vi "Test1.vi"   [LabVIEW 2020]
uses:
  MelsecMcNet/MelsecMcNet.lvclass
  lModbusRtu/ModbusRtu.lvclass
  InovanceTCP/InovanceModbusTcp.lvclass
  InovanceSerial/InovanceSerialModbusRtu.lvclass
  Abstract PLC Controler/Abs Controler.lvclass
  E:/Git/Libraries/develop/HslCommunication/Abstract PLC Controler/Abs Controler.lvclass
  E:/Git/Libraries/develop/HslCommunication/lModbusRtu/ModbusRtu.lvclass
  E:/Git/Libraries/develop/HslCommunication/MelsecMcNet/MelsecMcNet.lvclass
  E:/Git/Libraries/develop/HslCommunication/InovanceTCP/InovanceModbusTcp.lvclass
  E:/Git/Libraries/develop/HslCommunication/InovanceSerial/InovanceSerialModbusRtu.lvclass
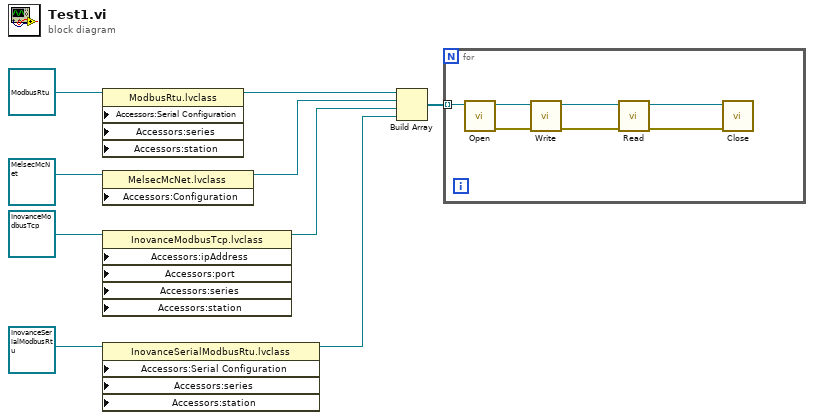
[diagram p0: block diagram]
diagram:
  n1 = property class="ModbusRtu.lvclass" props=["Accessors:Serial Configuration", "Accessors:series", "Accessors:station"](reference=refnum<class "ModbusRtu.lvclass"> refnum ("HslCommunication.lvlib:ModbusRtu.lvclass")) -> (reference out=w5:refnum<class "ModbusRtu.lvclass">)  [unwired: 4 in, 1 out]
  n2 = property class="MelsecMcNet.lvclass" props=["Accessors:Configuration"](reference=refnum<class "MelsecMcNet.lvclass"> refnum ("HslCommunication.lvlib:MelsecMcNet.lvclass")) -> (reference out=w3:refnum<class "MelsecMcNet.lvclass">)  [unwired: 2 in, 1 out]
  n3 = property class="InovanceModbusTcp.lvclass" props=["Accessors:ipAddress", "Accessors:port", "Accessors:series", "Accessors:station"](reference=refnum<class "InovanceModbusTcp.lvclass"> refnum ("HslCommunication.lvlib:InovanceModbusTcp.lvclass")) -> (reference out=w2:refnum<class "InovanceModbusTcp.lvclass">)  [unwired: 5 in, 1 out]
  n4 = property class="InovanceSerialModbusRtu.lvclass" props=["Accessors:Serial Configuration", "Accessors:series", "Accessors:station"](reference=refnum<class "InovanceSerialModbusRtu.lvclass"> refnum ("HslCommunication.lvlib:InovanceSerialModbusRtu.lvclass")) -> (reference out=w1:refnum<class "InovanceSerialModbusRtu.lvclass">)  [unwired: 4 in, 1 out]
  n5 = Build Array(w5, w3, w2, w1) -> (w4:refnum<class "Abs Controler.lvclass">[])
  n6 = for {
    tunnel: w4 -> [w10] mode=indexing
    n7 = call-dynamic "Open.vi"("MelsecTCP in"=w10) -> ("error out"=w11:errorcluster, "MelsecTCP out"=w12:refnum<class "Abs Controler.lvclass">)  [unwired: 9 in]
    n8 = call-dynamic "Write.vi"("error in (no error)"=w11, "MelsecTCP in"=w12) -> ("error out"=w15:errorcluster, "MelsecTCP out"=w16:refnum<class "Abs Controler.lvclass">)  [unwired: 8 in]
    n9 = call-dynamic "Read.vi"("error in (no error)"=w15, "MelsecTCP in"=w16) -> ("error out"=w13:errorcluster, "MelsecTCP out"=w14:refnum<class "Abs Controler.lvclass">)  [unwired: 7 in, 1 out]
    n10 = call-dynamic "Close.vi"("error in (no error)"=w13, "MelsecTCP in"=w14) -> ()  [unwired: 8 in, 2 out]
  }
